vi "待机状态数据存储写入和切换量程(子VI).vi"   [LabVIEW 2016, in "斯坦道CODMn.lvlib"]
uses:
  <vilib>/ptbypt/NI_PtbyPt.lvlib
types:
  T1 = cluster{"因子编码":u32, "单位":u16, "标样参考值":sgl, "水样数据时间":timestamp, "水样实测值":sgl, "水样数据标识":string, "标样数据时间":timestamp, "标样实测值":sgl, "标样数据标识":string, "空白数据时间":timestamp, "空白实测值":sgl, "空白数据标识":string, "零点核查数据时间":timestamp, "零点核查实测值":sgl, "零点核查数据标识":string, "跨度核查数据时间":timestamp, "跨度核查实测值":sgl, "跨度核查数据标识":string, "加标回收数据时间":timestamp, "加标回收实测值":sgl, "加标回收数据标识":string, "平行样数据时间":timestamp, "平行样实测值":sgl, "平行样数据标识":string}
  T2 = cluster{"时间":timestamp, "测量模式":string, "数据类型":string, "检测值":sgl, "单位":string, "数据标识":string, "因子编码":string, "标样参考值":sgl, "ORP-A":sgl, "ORP-B":sgl, "ORP-K":sgl, "COD滴定值":sgl, "高锰酸钾滴定数":sgl, "温度":sgl, "量程":sgl, "LastTime":timestamp, "序列号:":string, "跨度值":sgl}
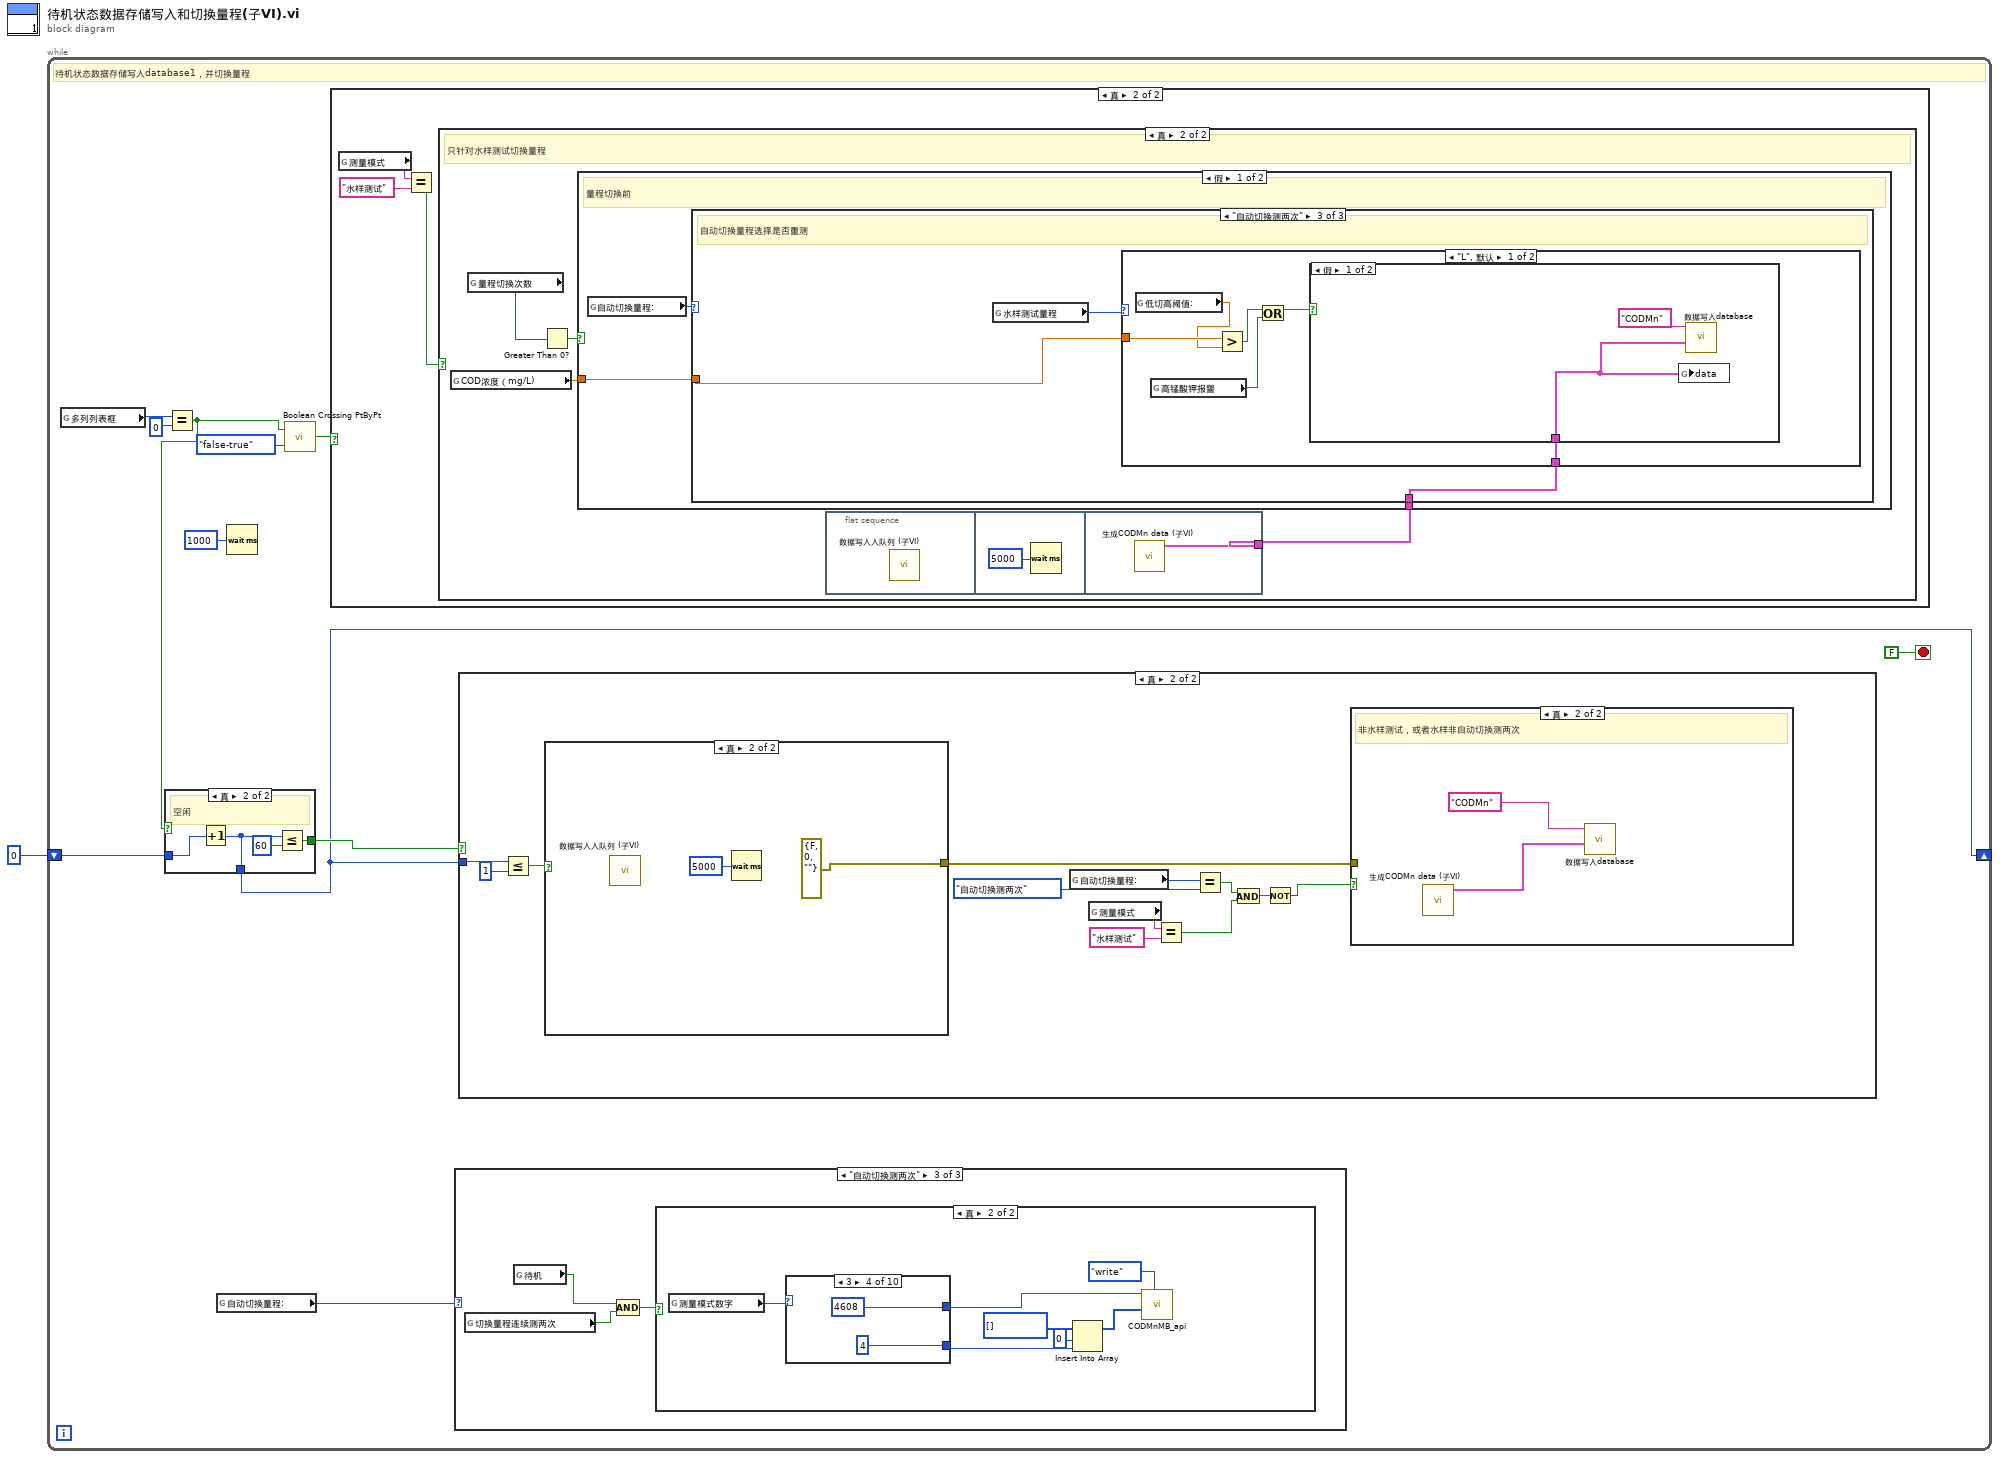
[diagram p0: block diagram]
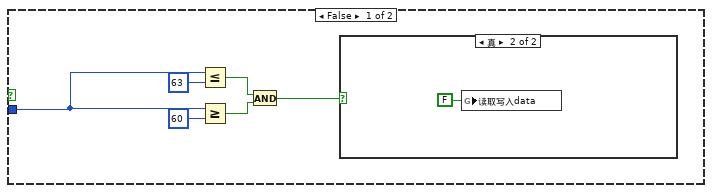
[diagram p2: hidden frame]
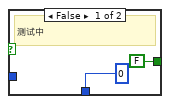
[diagram p6: hidden frame]
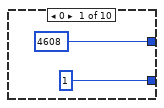
[diagram p10: hidden frame]
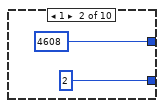
[diagram p11: hidden frame]
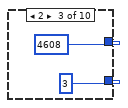
[diagram p12: hidden frame]
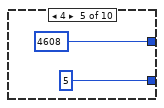
[diagram p13: hidden frame]
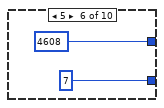
[diagram p14: hidden frame]
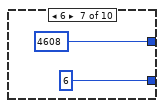
[diagram p15: hidden frame]
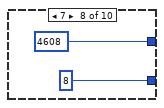
[diagram p16: hidden frame]
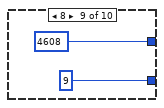
[diagram p17: hidden frame]
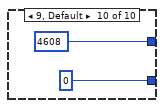
[diagram p18: hidden frame]
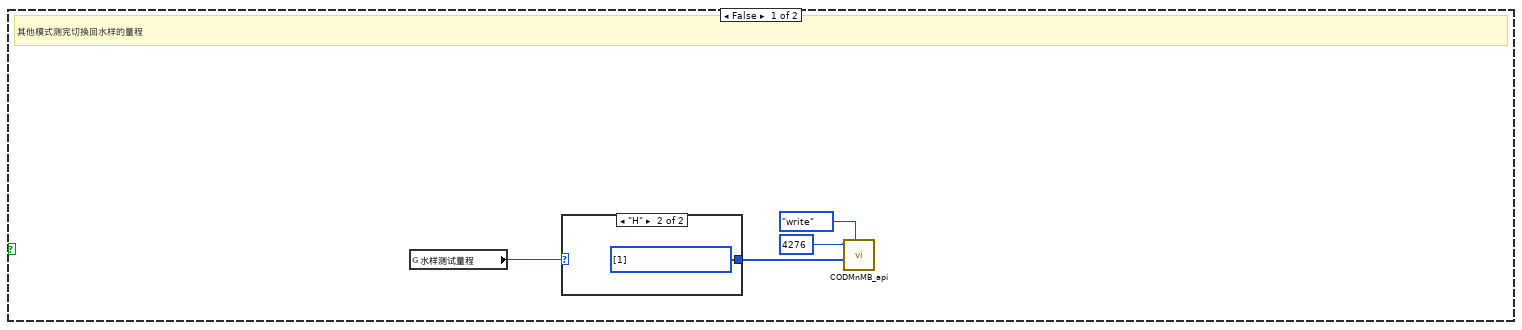
[diagram p20: hidden frame]
diagram:
  n1 = while {
    shift-right: [w2] -> _
    shift-left: 0 ("y") -> [w7]
    stop <- FALSE stop-if-true
    # "待机状态数据存储写入database1，并切换量程"
    n2 = global read "运行时序全局变量.vi" "多列列表框"() -> (w9:i32)
    n3 = Equal?(x=w9, y=0) -> (x = y?=w4:bool)
    n4 = case shown="真" w4 {
      tunnel: w7 -> [_ w40]
      tunnel: [0 w39] -> w2
      tunnel: [FALSE w38] -> w5
      frame False {
        # "测试中"
      }
      frame True {
        # "空闲"
        n5 = Increment(x=w40) -> (x+1=w39:i32)
        n6 = Less Or Equal?(x=w39, y=u32 60) -> (x <= y?=w38:bool)
      }
    }
    n7 = global read "CODMn断电保存全局变量.vi" "自动切换量程:"() -> (w8:enum16{"L", "H", "自动切换测一次", "自动切换测两次"})
    n8 = Wait (ms)(milliseconds to wait=u32 1000 ("等待时间（毫秒）")) -> ()  [unwired: 1 out]
    n9 = call <vilib>:"Boolean Crossing PtByPt.vi"("direction"=enum16{"either", "false-true", "true-false"}."false-true", "input"=w4) -> ("crossing"=w3:bool)  [unwired: 1 in]
    n10 = case shown="真" w3 {
      frame False {
      }
      frame True {
        n11 = global read "COD测量模式全局.vi" "测量模式"() -> (w74:string)
        n12 = Equal?(x=w74, y="水样测试") -> (x = y?=w72:bool)
        n13 = case shown="真" w72 {
          frame False {
            # "其他模式测完切换回水样的量程"
            n14 = global read "CODMn断电保存全局变量.vi" "水样测试量程"() -> (w75:enum16{"L", "H"})
            n15 = case shown="\"H\"" w75 {
              tunnel: [u16[] [0] ("values") u16[] [1] ("values")] -> w76
              frame "L", Default {
              }
              frame "H" {
              }
            }
            n16 = call "CODMnMB_api.vi"("STEP"=enum16{"open", "read", "write", "close"}."write", "values"=w76, "starting address"=u16 4276) -> ()  [unwired: 6 in, 3 out]
          }
          frame True {
            # "只针对水样测试切换量程"
            n17 = global read "COD浓度全局变量.vi" "COD浓度（mg/L)"() -> (w83:dbl)
            n18 = global read "COD内部交互全局.vi" "量程切换次数"() -> (w82:u8)
            n19 = Greater Than 0?(x=w82) -> (x > 0?=w84:bool)
            n20 = case shown="假" w84 {
              tunnel: w81 -> [w87 w139]
              tunnel: w83 -> [w89 _]
              frame False {
                # "量程切换前"
                n21 = global read "CODMn断电保存全局变量.vi" "自动切换量程:"() -> (w88:enum16{"L", "H", "自动切换测一次", "自动切换测两次"})
                n22 = case shown="\"自动切换测两次\"" w88 {
                  tunnel: w89 -> [_ w91 w115]
                  tunnel: w87 -> [_ _ w113]
                  frame "H", Default {
                    # "关闭自动切换量程"
                  }
                  frame "自动切换测一次" {
                    # "自动切换量程选择是否重测"
                    n23 = global read "CODMn断电保存全局变量.vi" "水样测试量程"() -> (w90:enum16{"L", "H"})
                    n24 = global read "COD测量模式全局.vi" "测量模式"() -> (w95:string)
                    n25 = Not Equal?(x=w95, y="水样测试") -> (x != y?=w93:bool)
                    n26 = case shown="真" w93 {
                      tunnel: [w110 w111] -> w92
                      tunnel: w91 -> [w110 _]
                      frame False {
                      }
                      frame True {
                        n27 = global read "CODMn断电保存全局变量.vi" "测量数据区"() -> (w112:T1)
                        n28 = Unbundle By Name(w112) -> ("水样实测值"=w111:sgl)
                      }
                    }
                    n29 = case shown="\"L\", 默认" w90 {
                      tunnel: w92 -> [w99 w105]
                      frame "L", Default {
                        n30 = global read "COD内部交互全局.vi" "高锰酸钾报警"() -> (w96:bool)
                        n31 = global read "CODMn断电保存全局变量.vi" "低切高阈值:"() -> (w97:dbl)
                        n32 = Greater?(x=w99, y=w97) -> (0:w100:bool)
                        n33 = Or(x=w96, y=w100) -> (x .or. y?=w98:bool)
                        n34 = case shown="真" w98 {
                          frame False {
                          }
                          frame True {
                            n35 = call "CODMnMB_api.vi"("STEP"=enum16{"open", "read", "write", "close"}."write", "values"=u16[] [1], "starting address"=u16 4276) -> ()  [unwired: 6 in, 3 out]
                          }
                        }
                      }
                      frame "H" {
                        n36 = global read "CODMn断电保存全局变量.vi" "高切低阈值:"() -> (w104:dbl)
                        n37 = Less?(x=w105, y=w104) -> (x < y?=w106:bool)
                        n38 = case shown="真" w106 {
                          frame False {
                          }
                          frame True {
                            n39 = call "CODMnMB_api.vi"("STEP"=enum16{"open", "read", "write", "close"}."write", "values"=u16[] [0], "starting address"=u16 4276) -> ()  [unwired: 6 in, 3 out]
                          }
                        }
                      }
                    }
                  }
                  frame "自动切换测两次" {
                    # "自动切换量程选择是否重测"
                    n40 = global read "CODMn断电保存全局变量.vi" "水样测试量程"() -> (w114:enum16{"L", "H"})
                    n41 = case shown="\"L\", 默认" w114 {
                      tunnel: w115 -> [w120 w130]
                      tunnel: w113 -> [w116 w128]
                      frame "L", Default {
                        n42 = global read "CODMn断电保存全局变量.vi" "低切高阈值:"() -> (w118:dbl)
                        n43 = global read "COD内部交互全局.vi" "高锰酸钾报警"() -> (w117:bool)
                        n44 = Greater?(x=w120, y=w118) -> (0:w121:bool)
                        n45 = Or(x=w121, y=w117) -> (x .or. y?=w119:bool)
                        n46 = case shown="假" w119 {
                          tunnel: w116 -> [w122 _]
                          frame False {
                            n47 = global write "COD内部交互全局.vi" "data"(w122) -> ()
                            n48 = call "数据写入database.vi"("data输入"=w122, "table"="CODMn") -> ()  [unwired: 9 in, 1 out]
                          }
                          frame True {
                            n49 = global write "COD内部交互全局.vi" "切换量程连续测两次"(TRUE ("切换量程连续测两次")) -> ()
                            n50 = call "CODMnMB_api.vi"("STEP"=enum16{"open", "read", "write", "close"}."write", "values"=u16[] [1], "starting address"=u16 4276) -> ()  [unwired: 6 in, 3 out]
                          }
                        }
                      }
                      frame "H" {
                        n51 = global read "CODMn断电保存全局变量.vi" "高切低阈值:"() -> (w129:dbl)
                        n52 = Less?(x=w130, y=w129) -> (x < y?=w131:bool)
                        n53 = case shown="真" w131 {
                          tunnel: w128 -> [w132 _]
                          frame False {
                            n54 = call "数据写入database.vi"("data输入"=w132, "table"="CODMn") -> ()  [unwired: 9 in, 1 out]
                          }
                          frame True {
                            # "重测第一次不存数据"
                            n55 = call "CODMnMB_api.vi"("STEP"=enum16{"open", "read", "write", "close"}."write", "values"=u16[] [0], "starting address"=u16 4276) -> ()  [unwired: 6 in, 3 out]
                            n56 = global write "COD内部交互全局.vi" "切换量程连续测两次"(TRUE ("切换量程连续测两次")) -> ()
                          }
                        }
                      }
                    }
                  }
                }
              }
              frame True {
                # "防止无限切量程"
                n57 = global write "COD内部交互全局.vi" "量程切换次数"(u8 0 ("量程切换次数")) -> ()
                n58 = call "数据写入database.vi"("data输入"=w139, "table"="CODMn") -> ()  [unwired: 9 in, 1 out]
              }
            }
            n59 = flat-sequence {
              tunnel: [w86] -> w81
              frame #0 {
                n60 = call "数据写入入队列 (子VI).vi"() -> ()  [unwired: 12 in]
              }
              frame #1 {
                n61 = Wait (ms)(milliseconds to wait=u32 5000 ("等待时间（毫秒）")) -> ()  [unwired: 1 out]
              }
              frame #2 {
                n62 = call "生成CODMn data (子VI).vi"() -> ("data"=w86:T2)  [unwired: 11 in]
              }
            }
          }
        }
      }
    }
    n63 = case shown="\"自动切换测两次\"" w8 {
      frame "H", Default {
      }
      frame "自动切换测一次" {
      }
      frame "自动切换测两次" {
        n64 = global read "COD内部交互全局.vi" "切换量程连续测两次"() -> (w43:bool)
        n65 = global read "COD内部交互全局.vi" "待机"() -> (w42:bool)
        n66 = Compound Arithmetic op=AND ("复合运算")(w42, w43) -> (w44:bool)
        n67 = case shown="真" w44 {
          frame False {
          }
          frame True {
            n68 = global read "COD内部交互全局.vi" "测量模式数字"() -> (w45:i32)
            n69 = case shown="3" w45 {
              tunnel: [u16 4608 ("address") u16 4608 ("address") u16 4608 ("address") u16 4608 ("address") u16 4608 ("address") u16 4608 ("address") u16 4608 ("address") u16 4608 ("address") u16 4608 ("address") u16 4608 ("address")] -> w46
              tunnel: [u16 1 ("address") u16 2 ("address") u16 3 ("address") u16 4 ("address") u16 5 ("address") u16 7 ("address") u16 6 ("address") u16 8 ("address") u16 9 ("address") u16 0 ("address")] -> w51
              frame 0 {
              }
              frame 1 {
              }
              frame 2 {
              }
              frame 3 {
              }
              frame 4 {
              }
              frame 5 {
              }
              frame 6 {
              }
              frame 7 {
              }
              frame 8 {
              }
              frame 9, Default {
              }
            }
            n70 = Insert Into Array(array=u16[] [] ("values"), index=0 ("索引"), new element=w51) -> (w47:u16[])
            n71 = call "CODMnMB_api.vi"("STEP"=enum16{"open", "read", "write", "close"}."write", "values"=w47, "starting address"=w46) -> ()  [unwired: 6 in, 3 out]
          }
        }
      }
    }
    n72 = case shown="真" w5 {
      tunnel: w2 -> [w15 w31]
      frame False {
        n73 = Less Or Equal?(x=w15, y=63) -> (x <= y?=w18:bool)
        n74 = Greater Or Equal?(x=w15, y=60) -> (x >= y?=w17:bool)
        n75 = And(x=w18, y=w17) -> (x .and. y?=w13:bool)
        n76 = case shown="真" w13 {
          frame False {
          }
          frame True {
            n77 = global write "COD内部交互全局.vi" "读取写入data"(FALSE ("读取写入data")) -> ()
          }
        }
      }
      frame True {
        n78 = Less Or Equal?(x=w31, y=1) -> (x <= y?=w29:bool)
        n79 = case shown="真" w29 {
          tunnel: [_ errorcluster {"status"=FALSE, "code"=0, "source"=""} ("错误常量")] -> w28
          frame False {
          }
          frame True {
            n80 = call "数据写入入队列 (子VI).vi"() -> ()  [unwired: 12 in]
            n81 = Wait (ms)(milliseconds to wait=u32 5000 ("等待时间（毫秒）")) -> ()  [unwired: 1 out]
          }
        }
        n82 = global read "CODMn断电保存全局变量.vi" "自动切换量程:"() -> (w25:enum16{"L", "H", "自动切换测一次", "自动切换测两次"})
        n83 = global read "COD测量模式全局.vi" "测量模式"() -> (w26:string)
        n84 = Equal?(x=w26, y="水样测试") -> (x = y?=w22:bool)
        n85 = Equal?(x=w25, y=enum16{"L", "H", "自动切换测一次", "自动切换测两次"}."自动切换测两次") -> (x = y?=w23:bool)
        n86 = And(x=w23, y=w22) -> (x .and. y?=w21:bool)
        n87 = Not(x=w21) -> (.not. x?=w20:bool)
        n88 = case shown="真" w20 {
          tunnel: w28 -> [_ _]
          frame False {
            # "自动切换测两次并且为水样测试"
          }
          frame True {
            # "非水样测试，或者水样非自动切换测两次"
            n89 = call "生成CODMn data (子VI).vi"() -> ("data"=w35:T2)  [unwired: 11 in]
            n90 = call "数据写入database.vi"("data输入"=w35, "table"="CODMn") -> ()  [unwired: 9 in, 1 out]
          }
        }
      }
    }
  }
